vi "simple_analog_scale.vi"(10 "Scale Const":T1, 11 "Analog":dbl) -> (3 "Units":dbl)   [LabVIEW 2013]
uses:
  scale_const.ctl
panel:
  # "Simple Analog Scale takes a number and linearl scales it between the scaling points\nWe use this for just about everything, including scaling analog inputs\nWe also use this VI to:\n-Scale the turret side-angle for the hood angle (fender shot)\n-Scale the error to linearly cap the integral term (PIFF gun speed controller)\n-Scale the new ball/old ball input (pct) to a gun speed"
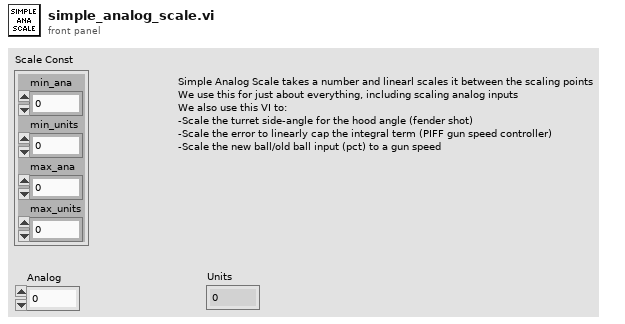
[diagram p1: front panel]
types:
  T1 = typedef "scale_const.ctl" = cluster{"min_ana":dbl, "min_units":dbl, "max_ana":dbl, "max_units":dbl}
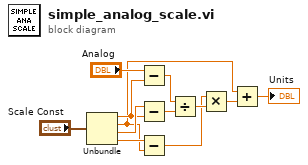
[diagram p0: block diagram]
diagram:
  n1 = Unbundle("Scale Const") -> ("min_ana"=w9:dbl, "min_units"=w1:dbl, "max_ana"=w10:dbl, "max_units"=w6:dbl)
  n2 = Subtract(x="Analog", y=w9) -> (x-y=w8:dbl)
  n3 = Subtract(x=w10, y=w9) -> (x-y=w7:dbl)
  n4 = Subtract(x=w6, y=w1) -> (x-y=w4:dbl)
  n5 = Divide(x=w8, y=w7) -> (x/y=w5:dbl)
  n6 = Multiply(x=w4, y=w5) -> (x*y=w2:dbl)
  n7 = Add(x=w1, y=w2) -> (x+y=→"Units":dbl)
